vi "test CRUD sample.vi"() -> ()   [LabVIEW 2019]
uses:
  <vilib>/httpClient/POSTBuffer.vi
  <vilib>/httpClient/LabVIEWHTTPClient.lvlib
panel:
  out "id":string[](array[string])
  in  "diameter":string
  in  "depth":string
  in  "height":string
  in  "weight":string
  in  "specimentno":string
  in  "Sample ID":string
  out "delete":string[](array[string])
  out "jobdesc":string[](array[string])
  out "jobno":string[](array[string])
  out "jobid":string[](array[string])
  out "status":string
  out "body":string
  in  "Sample No":string
  in  "Job Id":string
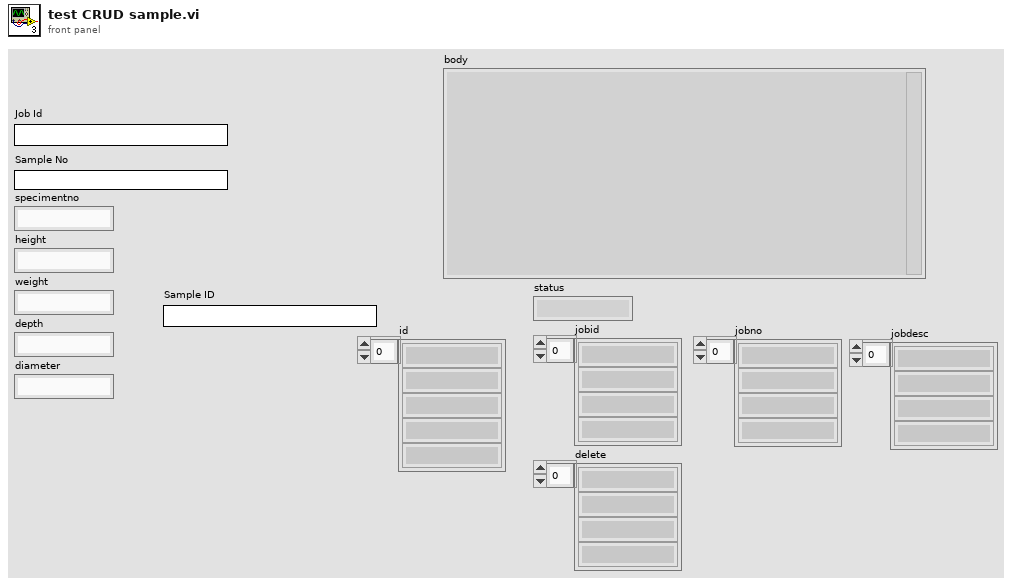
[diagram p1: front panel]
types:
  T1 = cluster{"action":string, "jobid":string, "sampleno":string, "specimentno":string, "weight":string, "height":string, "depth":string, "diameter":string}
  T2 = cluster{"action":string, "jobid":string, "sampleno":string, "specimentno":string, "weight":string, "height":string, "depth":string, "diameter":string, "id":string}
  T3 = cluster{"status":string, "data":cluster{"jobid":string, "sampleno":string, "specimentno":string, "weight":string, "height":string, "depth":string, "diameter":string, "delete":string, "id":string}[]}
  T4 = typedef "LabVIEWHTTPClient.lvlib/ClientHandle.ctl" = refnum<k1>
  T5 = cluster{"jobid":string, "sampleno":string, "specimentno":string, "weight":string, "height":string, "depth":string, "diameter":string, "delete":string, "id":string}[]
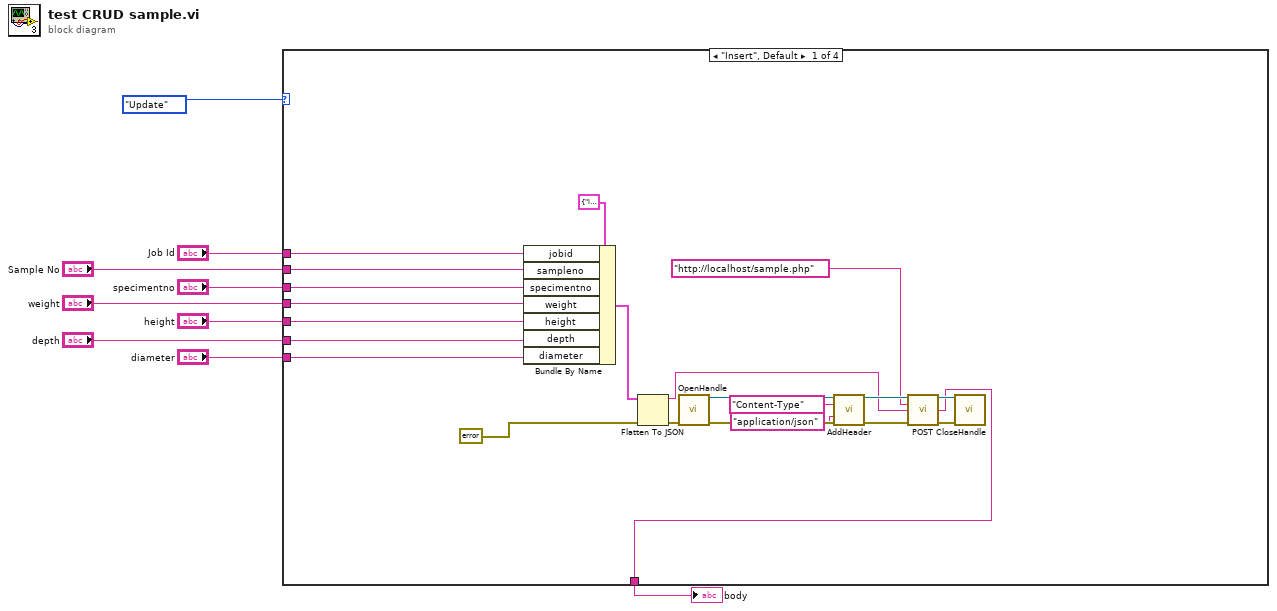
[diagram p0: block diagram]
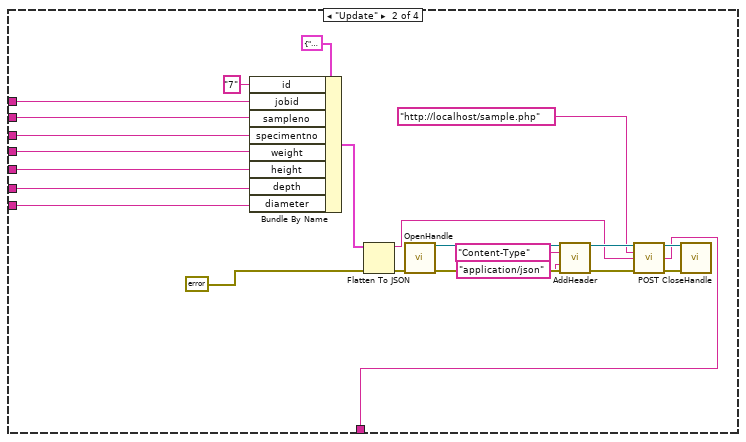
[diagram p2: hidden frame]
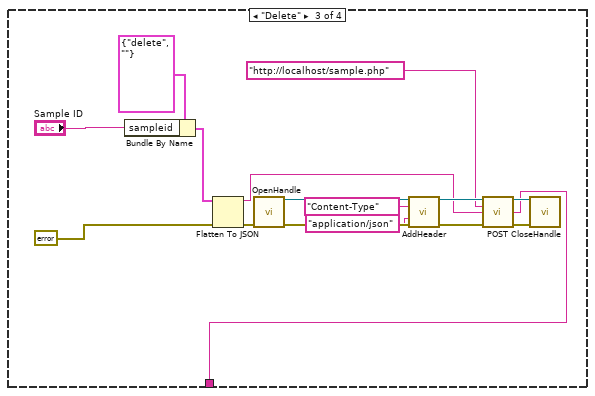
[diagram p3: hidden frame]
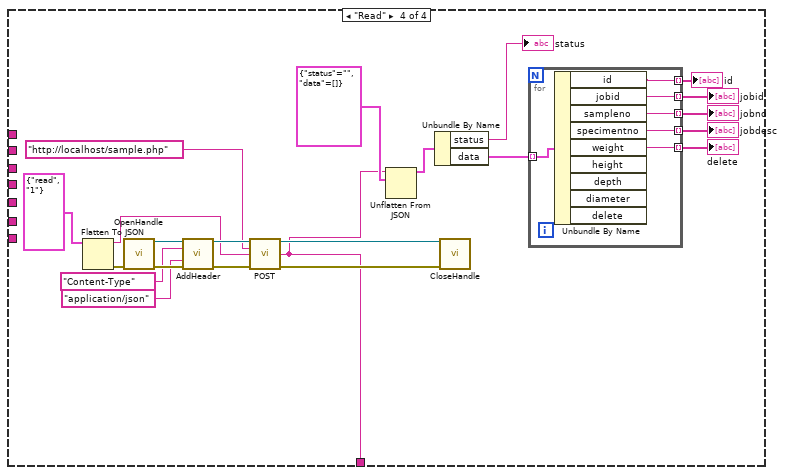
[diagram p4: hidden frame]
diagram:
  n1 = case shown="\"Insert\", Default" enum16{"Insert", "Read", "Delete", "Update"}."Update" {
    tunnel: [w17 w40 w55 w72] -> w8
    tunnel: "diameter" -> [w16 w33 _ _]
    tunnel: "depth" -> [w15 w34 _ _]
    tunnel: "height" -> [w14 w35 _ _]
    tunnel: "weight" -> [w13 w36 _ _]
    tunnel: "specimentno" -> [w12 w37 _ _]
    tunnel: "Sample No" -> [w11 w38 _ _]
    tunnel: "Job Id" -> [w10 w39 _ _]
    frame "Insert", Default {
      n2 = Bundle By Name(cluster=T1 {"action"="insert", "jobid"="", "sampleno"="", "specimentno"="", "weight"="", "height"="", "depth"="", "diameter"=""}, "jobid"=w10, "sampleno"=w11, "specimentno"=w12, "weight"=w13, "height"=w14, "depth"=w15, "diameter"=w16) -> (w19:T1)
      n3 = Flatten To JSON(anything=w19, error in (no error)=errorcluster {"status"=FALSE, "code"=0, "source"=""} ("error IO")) -> (JSON string=w18:string, 11:w20:errorcluster)  [unwired: 1 in]
      n4 = call <vilib>:"OpenHandle.vi"("error in (no error)"=w20) -> ("client handle out"=w27:T4, "error out"=w29:errorcluster)  [unwired: 13 in]
      n5 = call <vilib>:"AddHeader.vi"("client handle"=w27, "header"="Content-Type", "value"="application/json", "error in (no error)"=w29) -> ("client handle out"=w26:T4, "error out"=w28:errorcluster)  [unwired: 10 in]
      n6 = call-poly <vilib>:"POST.vi"("client handle"=w26, "url"="http://localhost/sample.php", "buffer"=w18, "error in (no error)"=w28) -> ("client handle out"=w21:T4, "body"=w17:string, "error out"=w22:errorcluster)  [unwired: 8 in, 1 out]
      n7 = call <vilib>:"CloseHandle.vi"("client handle"=w21, "error in (no error)"=w22) -> ()  [unwired: 13 in, 1 out]
    }
    frame "Update" {
      n8 = Bundle By Name(cluster=T2 {"action"="update", "jobid"="", "sampleno"="", "specimentno"="", "weight"="", "height"="", "depth"="", "diameter"="", "id"=""}, "id"="7", "jobid"=w39, "sampleno"=w38, "specimentno"=w37, "weight"=w36, "height"=w35, "depth"=w34, "diameter"=w33) -> (w42:T2)
      n9 = Flatten To JSON(anything=w42, error in (no error)=errorcluster {"status"=FALSE, "code"=0, "source"=""} ("error IO")) -> (JSON string=w41:string, 11:w43:errorcluster)  [unwired: 1 in]
      n10 = call <vilib>:"OpenHandle.vi"("error in (no error)"=w43) -> ("client handle out"=w50:T4, "error out"=w52:errorcluster)  [unwired: 13 in]
      n11 = call <vilib>:"AddHeader.vi"("client handle"=w50, "header"="Content-Type", "value"="application/json", "error in (no error)"=w52) -> ("client handle out"=w49:T4, "error out"=w51:errorcluster)  [unwired: 10 in]
      n12 = call-poly <vilib>:"POST.vi"("client handle"=w49, "url"="http://localhost/sample.php", "buffer"=w41, "error in (no error)"=w51) -> ("client handle out"=w44:T4, "body"=w40:string, "error out"=w45:errorcluster)  [unwired: 8 in, 1 out]
      n13 = call <vilib>:"CloseHandle.vi"("client handle"=w44, "error in (no error)"=w45) -> ()  [unwired: 13 in, 1 out]
    }
    frame "Delete" {
      n14 = Bundle By Name(cluster=cluster{"action":string, "sampleid":string} {"action"="delete", "sampleid"=""}, "sampleid"="Sample ID") -> (w57:cluster{"action":string, "sampleid":string})
      n15 = Flatten To JSON(anything=w57, error in (no error)=errorcluster {"status"=FALSE, "code"=0, "source"=""} ("error IO")) -> (JSON string=w56:string, 11:w58:errorcluster)  [unwired: 1 in]
      n16 = call <vilib>:"OpenHandle.vi"("error in (no error)"=w58) -> ("client handle out"=w65:T4, "error out"=w67:errorcluster)  [unwired: 13 in]
      n17 = call <vilib>:"AddHeader.vi"("client handle"=w65, "header"="Content-Type", "value"="application/json", "error in (no error)"=w67) -> ("client handle out"=w64:T4, "error out"=w66:errorcluster)  [unwired: 10 in]
      n18 = call-poly <vilib>:"POST.vi"("client handle"=w64, "url"="http://localhost/sample.php", "buffer"=w56, "error in (no error)"=w66) -> ("client handle out"=w59:T4, "body"=w55:string, "error out"=w60:errorcluster)  [unwired: 8 in, 1 out]
      n19 = call <vilib>:"CloseHandle.vi"("client handle"=w59, "error in (no error)"=w60) -> ()  [unwired: 13 in, 1 out]
    }
    frame "Read" {
      n20 = Flatten To JSON(anything=cluster{"action":string, "jobid":string} {"action"="read", "jobid"="1"}) -> (JSON string=w85:string, 11:w86:errorcluster)  [unwired: 2 in]
      n21 = call <vilib>:"OpenHandle.vi"("error in (no error)"=w86) -> ("client handle out"=w90:T4, "error out"=w92:errorcluster)  [unwired: 13 in]
      n22 = call <vilib>:"AddHeader.vi"("client handle"=w90, "header"="Content-Type", "value"="application/json", "error in (no error)"=w92) -> ("client handle out"=w89:T4, "error out"=w91:errorcluster)  [unwired: 10 in]
      n23 = call-poly <vilib>:"POST.vi"("client handle"=w89, "url"="http://localhost/sample.php", "buffer"=w85, "error in (no error)"=w91) -> ("client handle out"=w87:T4, "body"=w72:string, "error out"=w88:errorcluster)  [unwired: 8 in, 1 out]
      n24 = Unflatten From JSON(JSON string=w72, type and defaults=T3 {"status"="", "data"=[]}) -> (value=w79:T3)  [unwired: 5 in, 1 out]
      n25 = Unbundle By Name(w79) -> ("status"=→"status":string, "data"=w78:T5)
      n26 = call <vilib>:"CloseHandle.vi"("client handle"=w87, "error in (no error)"=w88) -> ()  [unwired: 13 in, 1 out]
      n27 = for {
        tunnel: w78 -> [w98] mode=indexing
        tunnel: [w97] -> w76 mode=indexing
        tunnel: [w96] -> w74 mode=indexing
        tunnel: [w95] -> w73 mode=indexing
        tunnel: [w94] -> w75 mode=indexing
        tunnel: [w93] -> w71 mode=indexing
        n28 = Unbundle By Name(w98) -> ("id"=w93:string, "jobid"=w97:string, "sampleno"=w96:string, "specimentno"=w95:string, "weight"=w94:string)  [unwired: 4 out]
      }
      "jobid" <- w76
      "jobno" <- w74
      "jobdesc" <- w73
      "delete" <- w75
      "id" <- w71
    }
  }
  "body" <- w8
